vi "Gui_SetupTimingScript_Ions.vi"(8 "error in (no error)":errorcluster, 11 "QMH UI Cluster":T4) -> (0 "error out":errorcluster caption="sortie d'erreur")   [LabVIEW 2018]
uses:
  controls/EXPERT_Inputs.ctl
  controls/DIGIT_5122_Inputs.ctl
  <instrlib>/niScope/Controls/niScope trigger source.ctl
  controls/HSDIO_6541_Inputs.ctl
  <instrlib>/niHSDIO/niHSDIO.llb/niHSDIO_ctl Trigger Source Values (Ring).ctl
  controls/SOFTWARE_Inputs.ctl
  controls/AO_6711_Inputs.ctl
  controls/AWG_5421_Inputs.ctl
  <instrlib>/niFgen/niFgen.llb/niFgen_ctl Trigger Source Values (Ring).ctl
  controls/XML_Inputs.ctl
  controls/SEQUENCE_Inputs.ctl
  controls/EXCIT_Inputs.ctl
  controls/DATA_Inputs.ctl
  controls/TIMING_Inputs.ctl
  controls/PROCESSING_Inputs.ctl
  controls/TRAPPING_Inputs.ctl
  controls/TIMING_Mandatory_Items.ctl
  controls/QMH_UI_Cluster.ctl
  controls/QMH_UI_References.ctl
  controls/QMH_UI_Report.ctl
  controls/QMH_UI_Command.ctl
  controls/QMH_ICR_Command.ctl
  controls/QMH_Status.ctl
  controls/TIMING_Table.ctl
  controls/TIMING_Optional_Items.ctl
panel:
  out "Ouput Script":string
  in  "TIMING Table":T1={"Mandatory Items"={"Script Name"="", "GINI Time Period"=100.0, "HSDIO Delay"=60.0, "Shutter Duration before"=50000.0, "Shutter Duration after"=50000.0, "Filter Tau"=2.0, "Emtyping Duration"=1000.0}, "Optional Items"={"Eject"=0, "Acq"=0, "Excit"=0, "Gas"=0, "Laser"=0, "Lamp"=0}, "Times Table"=[["Excit1", "name", "Swift", "0.5", "1200", "70", "150", "550", "0", "0", "0"]]} {"Optional Items"."Laser" min=0 max=3; "Optional Items"."Gas" min=0 max=5; "Mandatory Items"."GINI Time Period" min=100000.0 max=1000000.0 format="%#_7g"; "Mandatory Items"."Shutter Duration after" min=2.0 max=100000.0; "Mandatory Items"."HSDIO Delay" min=0.0 max=100.0; "Mandatory Items"."Shutter Duration before" min=2.0 max=100000.0; "Mandatory Items"."Filter Tau" min=1000.0 max=2000.0; "Mandatory Items"."Emtyping Duration" min=2.0 format="%#_8g"}
  out "Total Duration (estimation)":i16=1 min=1 max=10 step=1
  in  "Number of Ions Refills":i16=1 min=1 max=100 step=1
  in  "REWRITE HEADER":bool
  in  "Mandatory Items":T2={"Script Name"="ForTestPurpose", "GINI Time Period"=100.0, "HSDIO Delay"=60.0, "Shutter Duration before"=50000.0, "Shutter Duration after"=50000.0, "Filter Tau"=2000.0, "Emtyping Duration"=1000000.0} caption="TIMING Mandatory Items" {"GINI Time Period" min=100000.0 max=1000000.0 format="%#_7g"; "Shutter Duration after" min=2.0 max=100000.0; "HSDIO Delay" min=0.0 max=100.0; "Shutter Duration before" min=2.0 max=100000.0; "Filter Tau" min=1000.0 max=2000.0; "Emtyping Duration" min=2.0 format="%#_8g"}
  in  "SEQUENCE Inputs":T10={"EXCIT Inputs"={"Number of Excitations"=1, "Script Text"="", "Table of Waveforms"=[]}, "DATA Inputs"={"Record Length"=524000, "Sample Rate"=2000000.0, "Data Type"=0, "Vertical Range"=10.0, "Acquisition Duration"=262.0}, "TIMING Inputs"={"Number of Acquisitions "=1, "Number of Accumulations"=1, "Table of Waveforms"=[], "Script Text"=""}, "PROCESSING Inputs"={"Reference Mass"=300.0939, "Cyclotron Freq"=255.727, "Magnetron Freq"=0.001}, "TRAPPING Inputs"={"Number of Channels"=4, "Init Values"=[2.0, 9.0, 2.0, 9.0], "Opening Values"=[0.0, 0.0, 0.0, 0.0], "Trapping Values"=[2.0, 9.0, 2.0, 9.0], "Emptying Values"=[-10.0, -10.0, -10.0, -10.0], "Adiabatic ON"=FALSE, "Adiabatic Duration"=100, "Adiabatic Waveforms"=["Adiabatic_None_2_2_2000", "Adiabatic_Ramp_9_0_2000", "Adiabatic_None_2_2_2000", "Adiabatic_RC_9_0_2000"], "Ions Refill ON"=FALSE, "Number of Ions Refills"=1, "Trapping Delay"=400.0, "Trapping Duration"=300.0}} {"TRAPPING Inputs"."Trapping Duration" min=2.0; "TRAPPING Inputs"."Trapping Delay" min=2.0; "TRAPPING Inputs"."Number of Ions Refills" min=1 max=1000; "TRAPPING Inputs"."Trapping Values" min=-10.0 max=10.0; "TRAPPING Inputs"."Init Values" min=-10.0 max=10.0; "TRAPPING Inputs"."Emptying Values" min=-10.0 max=10.0; "TRAPPING Inputs"."Opening Values" min=-10.0 max=10.0; "PROCESSING Inputs"."Magnetron Freq" format="%.5g"; "PROCESSING Inputs"."Cyclotron Freq" format="%.5g"; "PROCESSING Inputs"."Reference Mass" format="%.5g"; "TIMING Inputs"."Number of Accumulations" min=0 max=50 step=1; "TIMING Inputs"."Number of Acquisitions" min=1 max=10 step=1; "DATA Inputs"."Vertical Range" items=["0.2"=0.2, "0.4"=0.4, "1"=1.0, "2"=2.0, "4"=4.0, "10"=10.0]; "DATA Inputs"."Data Type" items=["I16", "DBL"]; "DATA Inputs"."Sample Rate" items=["1 MHz"=1000000.0, "2 MHz"=2000000.0, "5 MHz"=5000000.0, "10 MHz"=10000000.0, "20 MHz"=20000000.0, "25 MHz"=25000000.0, "50 MHz"=50000000.0, "100 MHz"=100000000.0]; "EXCIT Inputs"."Number of Excitations" min=1 max=10}
  out "Number of Excitations":i16=1 min=1 max=10 step=1
  in  "Number Of Accumulations":i16=1 caption="Number of Accumulations" min=0 max=50 step=1
  out "Number of Acquisitions":i16=1 min=1 max=10 step=1
  in  "OK":bool
  in  "CHECK":bool
  in  "EXPERT Inputs":T16={"DIGIT 5122 Inputs"={"Sample Rate"=10000.0, "Resource Name"="DIGIT_5122", "Channel Name"="0", "Trigger Source"="VAL_EXTERNAL", "Vertical Range"=10.0, "Trigger Level"=3.0}, "HSDIO 6541 Inputs"={"Resource Name"="HSDIO_6541", "Clock Rate"=1000000.0, "Trigger Source"="PFI0"}, "SOFTWARE Inputs"={"Application Directory"=path "D:/S.O.F.T.S/LABVIEW/PIL", "Software Version"="1.0.0", "Data Path"=path "D:/PIRENEA/DATA", "XML Path"=path "D:/PIRENEA/DATA", "XML File Filter"="*.xml", "XML Saved Path"=path "D:/PIRENEA/DATA/SAVED", "Excit Scripts Path"=path "D:/PIRENEA/EXCIT_SCRIPTS", "Excit Scripts File Filter"="*.txt", "Excit Waveforms Path"=path "D:/PIRENEA/EXCIT_WFMS", "Excit Waveforms File Filter"="*.bin", "Timing Scripts Path"=path "D:/PIRENEA/TECHNICAL/TIMING_SCRIPTS", "Timing Scripts File Filter"="*.txt", "Timing Waveforms Path"=path "D:/PIRENEA/TECHNICAL/TIMING_WFMS", "Timing Waveforms File Filter"="*.bin", "Trapping Waveforms Path"=path "D:/PIRENEA/TRAPPING_WFMS", "Trapping Waveforms File Filter"="*.bin"}, "AO 6711 Inputs"={"Physical Channels"="AO_6711/ao0:3", "Min Voltage"=-10.0, "Max Voltage"=10.0, "Trigger Source"="/AO_6711/PFI3", "Counter"="AO_6711/ctr0"}, "AWG 5421 Inputs"={"Resource Name"="AWG_5421", "Sample Rate"=10000000.0, "Trigger Type"=2, "Trigger Source"="PFI0", "Waveform Gain"=0.31, "Digital Filter ON"=TRUE}, "XML Inputs"={"Version Tag Name"="XML_Version", "Version String"="1.0"}} {"AWG 5421 Inputs"."Sample Rate" format="%.2p"; "AWG 5421 Inputs"."Trigger Type" items=["None", "Software Edge", "Digital Edge", "Digital Level"]; "AO 6711 Inputs"."Max Voltage" min=-10.0 max=10.0; "AO 6711 Inputs"."Min Voltage" min=-10.0 max=10.0; "HSDIO 6541 Inputs"."Clock Rate" format="%.2p"; "DIGIT 5122 Inputs"."Trigger Level" format="%.2f"; "DIGIT 5122 Inputs"."Vertical Range" format="%.2f"; "DIGIT 5122 Inputs"."Sample Rate" step=65535.0 format="%#_3p"}
  in  "LOAD":bool
  in  "Timing Script":string
  # "GO_out"
  # "Gout"
  # "GI_in"
  # "Gin"
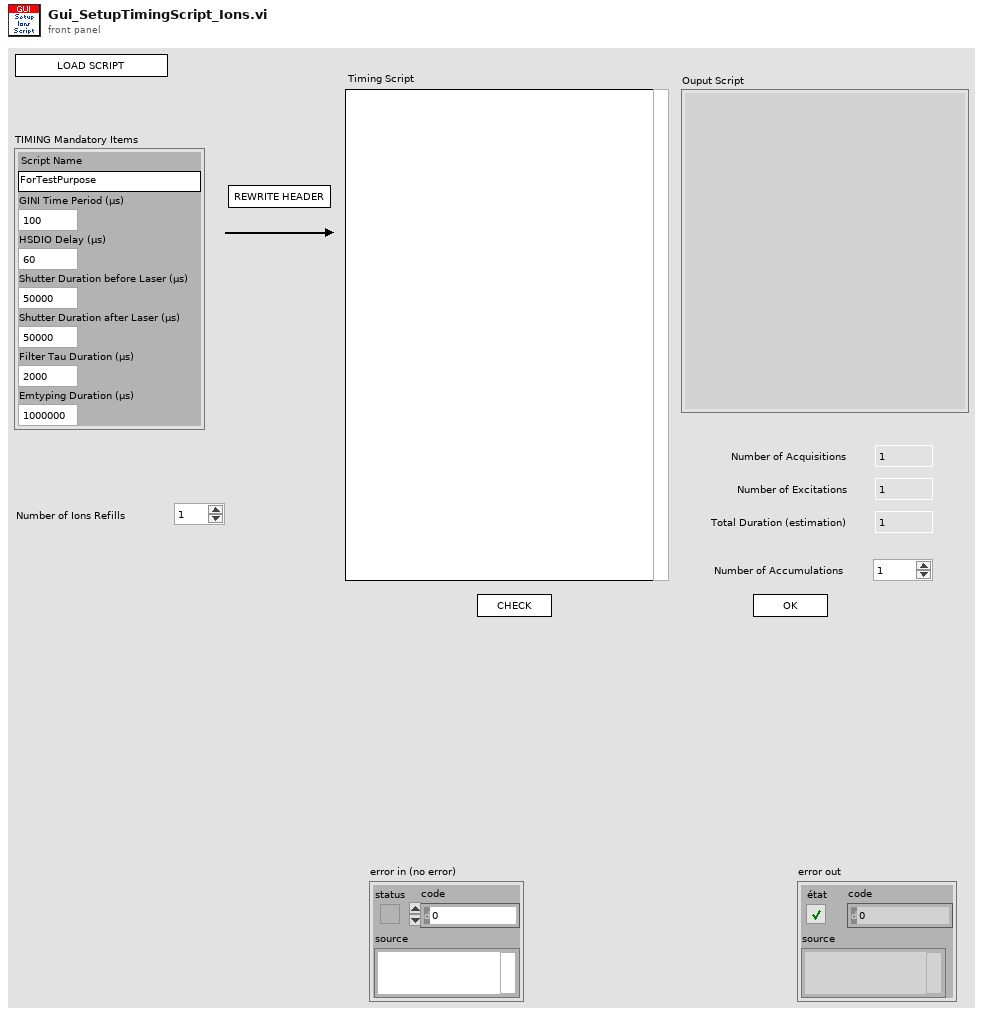
[diagram p1: front panel]
types:
  T1 = typedef "TIMING_Table.ctl" = cluster{"Mandatory Items":T2, "Optional Items":T3, "Times Table":string[][]}
  T2 = typedef "TIMING_Mandatory_Items.ctl" = cluster{"Script Name":string, "GINI Time Period":dbl, "HSDIO Delay":dbl, "Shutter Duration before":dbl, "Shutter Duration after":dbl, "Filter Tau":dbl, "Emtyping Duration":dbl}
  T3 = typedef "TIMING_Optional_Items.ctl" = cluster{"Eject":u32, "Acq":i32, "Excit":u32, "Gas":i32, "Laser":i32, "Lamp":i32}
  T4 = typedef "QMH_UI_Cluster.ctl" = cluster{"QMH UI References":T5, "QMH UI Report":T6}
  T5 = typedef "QMH_UI_References.ctl" = cluster{"Refnum Load":refnum<vi>, "Refnum Save As":refnum<vi>, "Refnum Start":refnum<vi>, "Refnum Exit":refnum<vi>, "Refnum Tabs":refnum<vi>, "Refnum SPECTRUM":refnum<vi>, "Refnum EXPERIMENT":refnum<vi>, "Refnum VOLTAGES":refnum<vi>, "Refnum SEQUENCE":refnum<vi>, "Refnum EXPERT":refnum<vi>, "Refnum EXCIT Table":refnum<vi>, "Refnum TIMING Table":refnum<vi>, "Refnum CHANGE Experiment":refnum<vi>, "Refnum CHANGE Voltages":refnum<vi>, "Refnum CHANGE Sequence":refnum<vi>, "Refnum CHANGE Expert":refnum<vi>, "Refnum CHANGE Scientist":refnum<vi>, "Refnum PIL Status":refnum<vi>}
  T6 = typedef "QMH_UI_Report.ctl" = cluster{"UI Status":T7, "ICR Status":T8, "QMH Status":T9}
  T7 = typedef "QMH_UI_Command.ctl" = enum16{"Initialize", "UI Load", "UI Save", "UI Save As", "UI Change Experiment", "UI Change Voltages", "UI Change Sequence", "UI Change Expert", "UI Change Scientist", "Ready to Start", "UI Start", "Waiting for ICR", "UI Exit", "Update Report", "Update ICR Status", "Waiting for User"}
  T8 = typedef "QMH_ICR_Command.ctl" = enum16{"Initialize", "Sequence Setup", "ICR Start", "ICR Stop", "Hardware Setup", "Next Accumulation", "Waiting for Trigger", "Sequence Started", "Sequence Finished", "Writing Data", "Hardware Reset", "Exit"}
  T9 = typedef "QMH_Status.ctl" = enum16{"Init", "Loading", "Setup", "Ready to Start", "Started", "Idle"}
  T10 = typedef "SEQUENCE_Inputs.ctl" = cluster{"EXCIT Inputs":T11, "DATA Inputs":T12, "TIMING Inputs":T13, "PROCESSING Inputs":T14, "TRAPPING Inputs":T15}
  T11 = typedef "EXCIT_Inputs.ctl" = cluster{"Number of Excitations":i32, "Script Text":string, "Table of Waveforms":string[]}
  T12 = typedef "DATA_Inputs.ctl" = cluster{"Record Length":i32, "Sample Rate":dbl, "Data Type":u8, "Vertical Range":dbl, "Acquisition Duration":dbl}
  T13 = typedef "TIMING_Inputs.ctl" = cluster{"Number of Acquisitions ":i16, "Number of Accumulations":i16, "Table of Waveforms":string[], "Script Text":string}
  T14 = typedef "PROCESSING_Inputs.ctl" = cluster{"Reference Mass":dbl, "Cyclotron Freq":dbl, "Magnetron Freq":dbl}
  T15 = typedef "TRAPPING_Inputs.ctl" = cluster{"Number of Channels":i32, "Init Values":dbl[], "Opening Values":dbl[], "Trapping Values":dbl[], "Emptying Values":dbl[], "Adiabatic ON":bool, "Adiabatic Duration":i32, "Adiabatic Waveforms":string[], "Ions Refill ON":bool, "Number of Ions Refills":i32, "Trapping Delay":dbl, "Trapping Duration":dbl}
  T16 = typedef "EXPERT_Inputs.ctl" = cluster{"DIGIT 5122 Inputs":T17, "HSDIO 6541 Inputs":T19, "SOFTWARE Inputs":T21, "AO 6711 Inputs":T22, "AWG 5421 Inputs":T23, "XML Inputs":T25}
  T17 = typedef "DIGIT_5122_Inputs.ctl" = cluster{"Sample Rate":dbl, "Resource Name":refnum<k15>, "Channel Name":string, "Trigger Source":T18, "Vertical Range":dbl, "Trigger Level":dbl}
  T18 = typedef "niScope trigger source.ctl" = string
  T19 = typedef "HSDIO_6541_Inputs.ctl" = cluster{"Resource Name":refnum<k15>, "Clock Rate":dbl, "Trigger Source":T20}
  T20 = typedef "niHSDIO_ctl Trigger Source Values (Ring).ctl" = string
  T21 = typedef "SOFTWARE_Inputs.ctl" = cluster{"Application Directory":path, "Software Version":string, "Data Path":path, "XML Path":path, "XML File Filter":string, "XML Saved Path":path, "Excit Scripts Path":path, "Excit Scripts File Filter":string, "Excit Waveforms Path":path, "Excit Waveforms File Filter":string, "Timing Scripts Path":path, "Timing Scripts File Filter":string, "Timing Waveforms Path":path, "Timing Waveforms File Filter":string, "Trapping Waveforms Path":path, "Trapping Waveforms File Filter":string}
  T22 = typedef "AO_6711_Inputs.ctl" = cluster{"Physical Channels":tag, "Min Voltage":dbl, "Max Voltage":dbl, "Trigger Source":tag, "Counter":tag}
  T23 = typedef "AWG_5421_Inputs.ctl" = cluster{"Resource Name":refnum<k15>, "Sample Rate":dbl, "Trigger Type":u16, "Trigger Source":T24, "Waveform Gain":dbl, "Digital Filter ON":bool}
  T24 = typedef "niFgen_ctl Trigger Source Values (Ring).ctl" = string
  T25 = typedef "XML_Inputs.ctl" = cluster{"Version Tag Name":string, "Version String":string}
  T26 = enum16{"Native", "Native Command Line", "UNIX", "Macintosh", "DOS"}
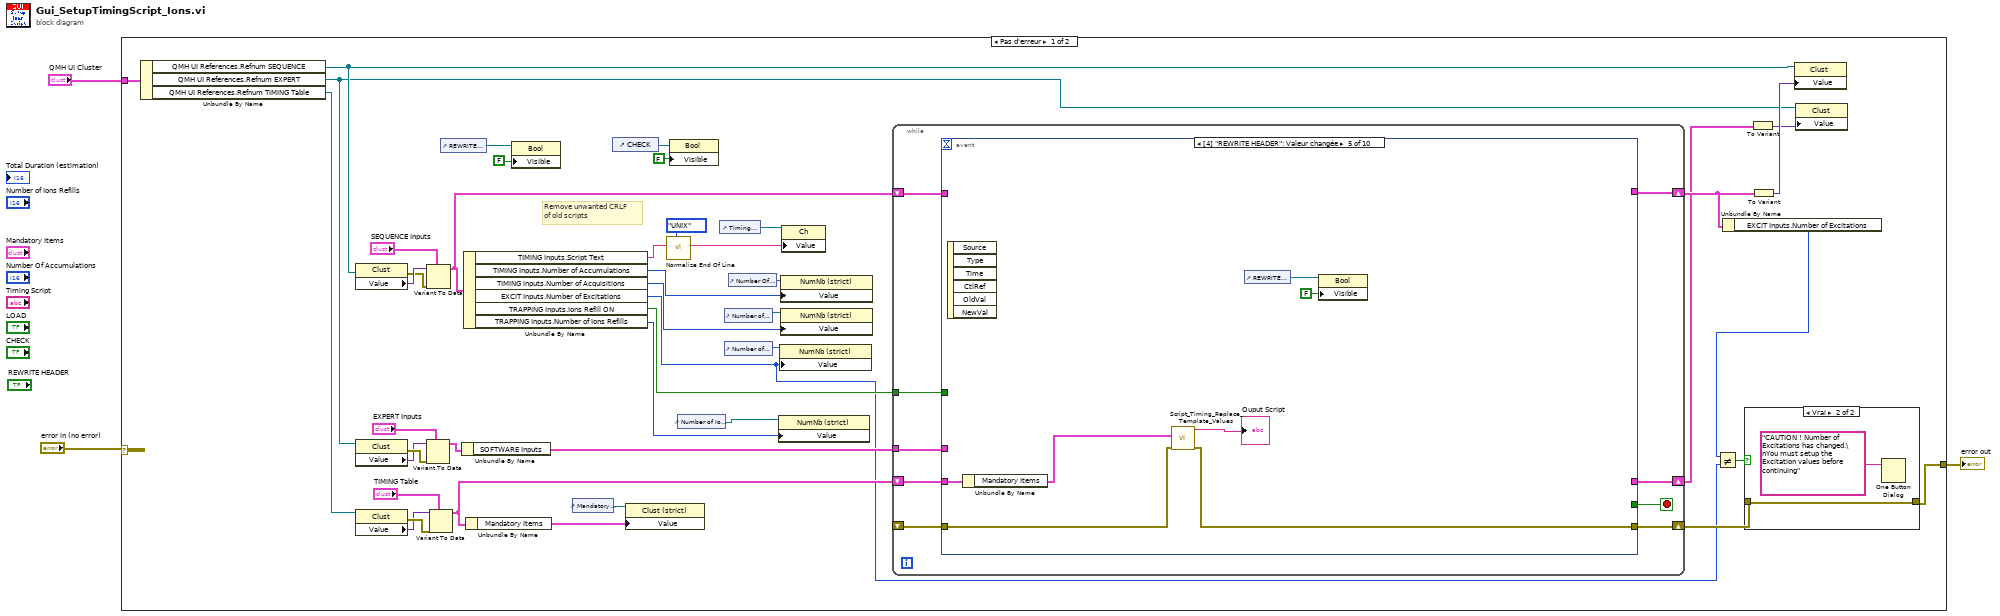
[diagram p0: block diagram]
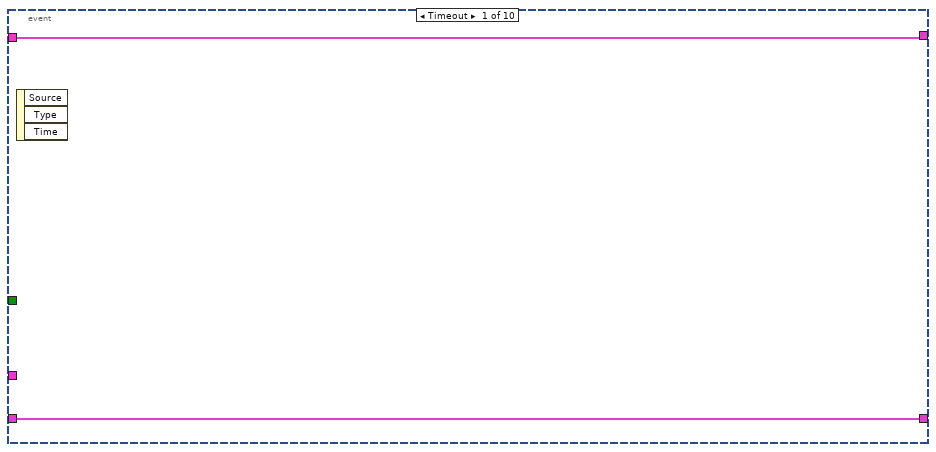
[diagram p3: hidden frame]
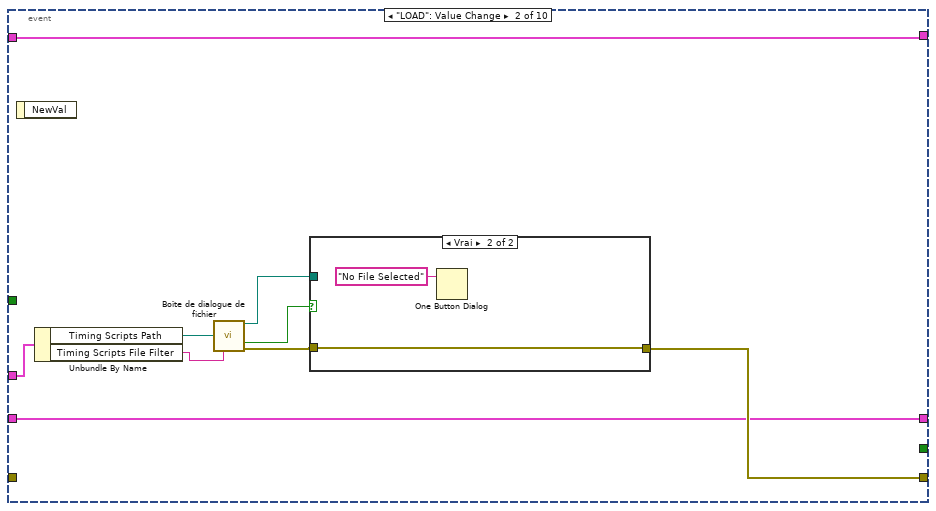
[diagram p4: hidden frame]
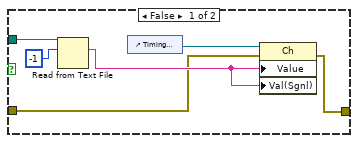
[diagram p5: hidden frame]
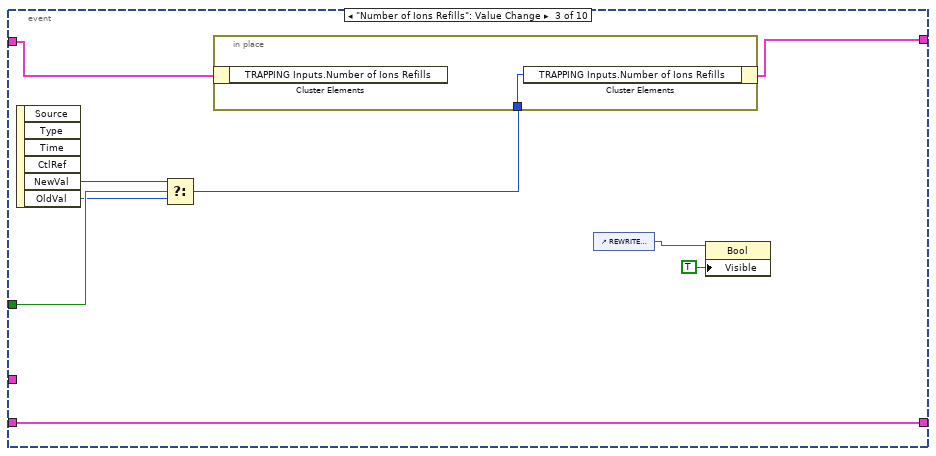
[diagram p6: hidden frame]
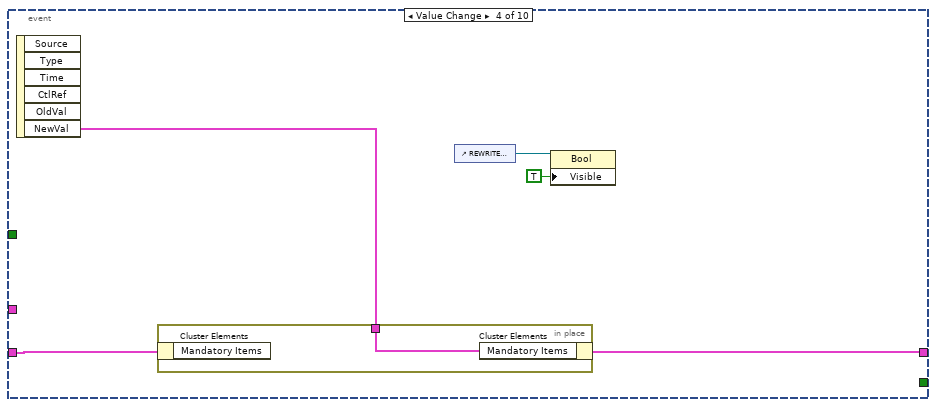
[diagram p7: hidden frame]
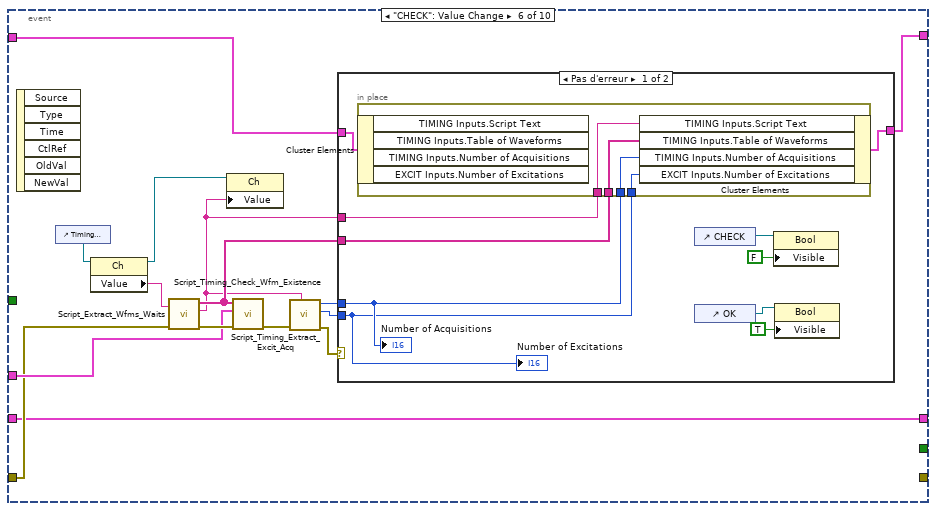
[diagram p8: hidden frame]
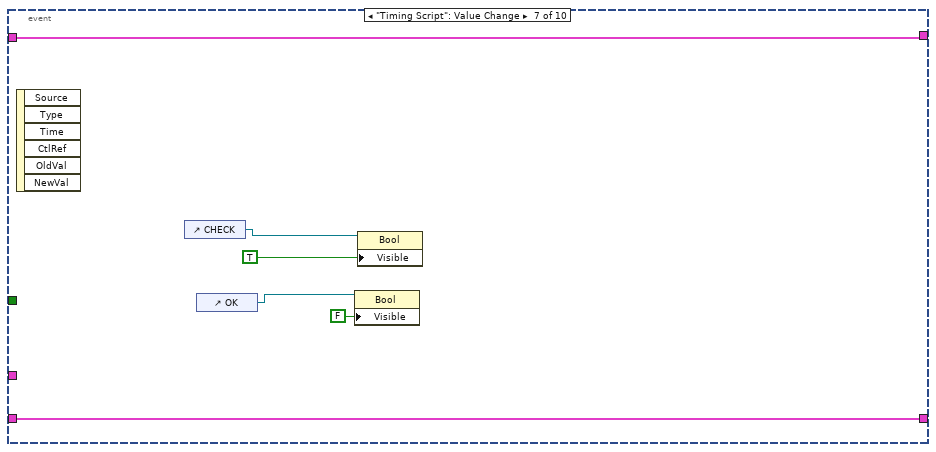
[diagram p10: hidden frame]
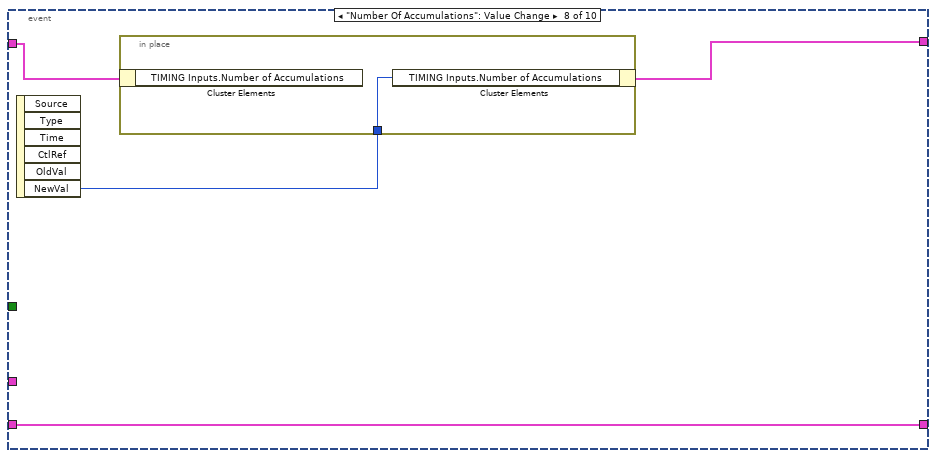
[diagram p11: hidden frame]
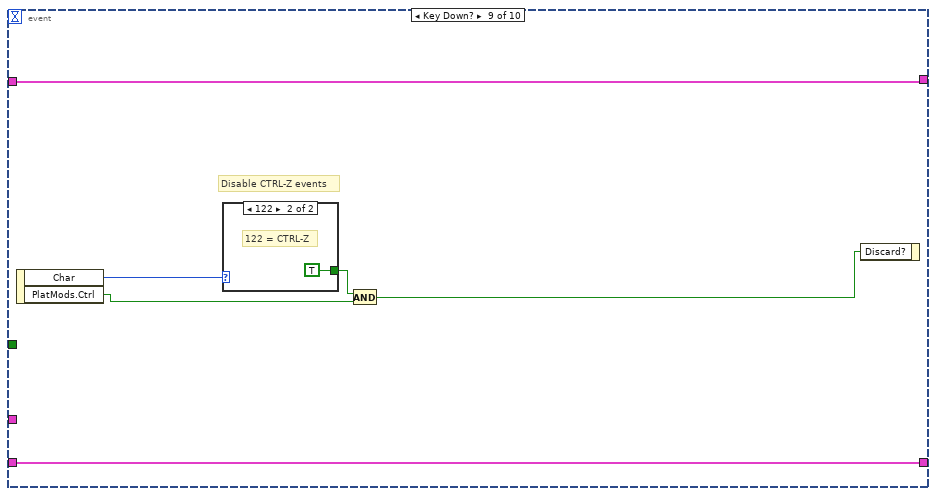
[diagram p12: hidden frame]
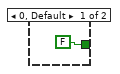
[diagram p13: hidden frame]
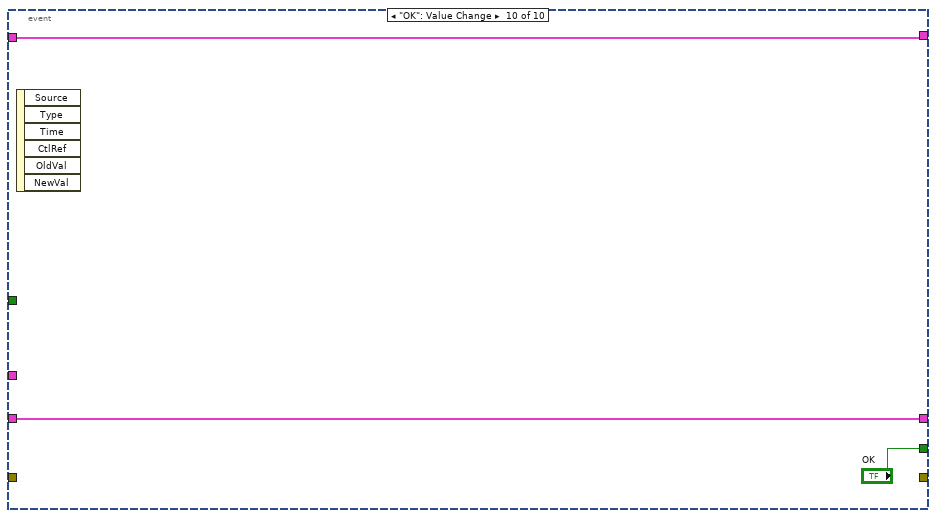
[diagram p14: hidden frame]
diagram:
  n1 = case shown="Pas d'erreur" "error in (no error)" {
    selector: "error in (no error)" -> [_ w154]
    tunnel: [w37 w154] -> w2
    tunnel: "QMH UI Cluster" -> [w34 _]
    frame No Error {
      # "Remove unwanted CRLF\nof old scripts"
      n2 = Unbundle By Name(w34) -> ("QMH UI References.Refnum SEQUENCE"=w14:refnum<vi>, "QMH UI References.Refnum EXPERT"=w7:refnum<vi>, "QMH UI References.Refnum TIMING Table"=w22:refnum<vi>)
      n3 = property class="Clust"(reference=w14) -> (error out=w15:errorcluster, "Value"=w33:variant)  [unwired: 1 in, 1 out]
      n4 = property class="Clust"(reference=w7) -> (error out=w27:errorcluster, "Value"=w24:variant)  [unwired: 1 in, 1 out]
      n5 = property class="Clust"(reference=w22) -> (error out=w26:errorcluster, "Value"=w25:variant)  [unwired: 1 in, 1 out]
      n6 = Variant To Data(error in=w27, type="EXPERT Inputs", Variant=w24) -> (data=w40:T16)  [unwired: 1 out]
      n7 = Variant To Data(error in=w15, type="SEQUENCE Inputs", Variant=w33) -> (data=w18:T10)  [unwired: 1 out]
      n8 = Variant To Data(error in=w26, type="TIMING Table", Variant=w25) -> (data=w13:T1)  [unwired: 1 out]
      n9 = control-ref of="REWRITE HEADER"() -> (w5:refnum<vi>)
      n10 = Unbundle By Name(w40) -> ("SOFTWARE Inputs"=w46:T21)
      n11 = Unbundle By Name(w18) -> ("TIMING Inputs.Script Text"=w31:string, "TIMING Inputs.Number of Accumulations"=w30:i16, "TIMING Inputs.Number of Acquisitions"=w29:i16, "EXCIT Inputs.Number of Excitations"=w9:i32, "TRAPPING Inputs.Ions Refill ON"=w10:bool, "TRAPPING Inputs.Number of Ions Refills"=w11:i32)
      n12 = Unbundle By Name(w13) -> ("Mandatory Items"=w20:T2)
      n13 = property class="Bool"(reference=w5, "Visible"=FALSE) -> ()  [unwired: 1 in, 2 out]
      n14 = control-ref of="Mandatory Items"() -> (w21:refnum<vi>)
      n15 = control-ref of="CHECK"() -> (w44:refnum<vi>)
      n16 = property class="Clust (strict)"(reference=w21, "Value"=w20) -> ()  [unwired: 1 in, 2 out]
      n17 = call <vilib>:"Normalize End Of Line.vi"("end of line (Native)"=T26."UNIX", "string in"=w31) -> ("string out"=w35:string)  [unwired: 6 in]
      n18 = property class="Bool"(reference=w44, "Visible"=FALSE) -> ()  [unwired: 1 in, 2 out]
      n19 = control-ref of="Number of Ions Refills"() -> (w12:refnum<vi>)
      n20 = control-ref of="Timing Script"() -> (w47:refnum<vi>)
      n21 = control-ref of="Number of Acquisitions"() -> (w42:refnum<vi>)
      n22 = control-ref of="Number of Excitations"() -> (w41:refnum<vi>)
      n23 = control-ref of="Number Of Accumulations"() -> (w43:refnum<vi>)
      n24 = property class="NumNb (strict)"(reference=w12, "Value"=w11) -> ()  [unwired: 1 in, 2 out]
      n25 = property class="NumNb (strict)"(reference=w41, "Value"=w9) -> ()  [unwired: 1 in, 2 out]
      n26 = property class="NumNb (strict)"(reference=w43, "Value"=w30) -> ()  [unwired: 1 in, 2 out]
      n27 = property class="NumNb (strict)"(reference=w42, "Value"=w29) -> ()  [unwired: 1 in, 2 out]
      n28 = property class="Ch"(reference=w47, "Value"=w35) -> ()  [unwired: 1 in, 2 out]
      n29 = while {
        shift-right: [w57] -> w38
        shift-left: _ -> [w59]
        tunnel: w46 -> [w54]
        shift-right: [w55] -> w17
        shift-left: w18 -> [w56]
        shift-right: [w51] -> w8
        shift-left: w13 -> [w53]
        tunnel: w10 -> [w52]
        stop <- w58 stop-if-true
        n30 = event shown="[4] \"REWRITE HEADER\": Valeur changée" {
          selector: _ -> [_ _ _ _ _ _ _ _ _ _]
          dyn-events: _ -> [_ _ _ _ _ _ _ _ _ _]
          timeout: _ -> [_ _ _ _ _ _ _ _ _ _]
          tunnel: w59 -> [_ _ _ _ w99 w103 _ _ _ _]
          tunnel: [_ w66 _ _ w98 _ _ _ _ _] -> w57
          tunnel: [_ _ _ _ _ _ _ _ _ "OK"] -> w58
          tunnel: w56 -> [w61 w67 w87 _ _ w114 w135 w139 w144 w152]
          tunnel: [w61 w67 w86 _ _ w113 w135 w140 w144 w152] -> w55
          tunnel: w54 -> [_ w65 _ _ _ w111 _ _ _ _]
          tunnel: w53 -> [w60 w62 w81 w93 w97 w102 w132 w138 w143 w151]
          tunnel: w52 -> [_ _ w85 _ _ _ _ _ _ _]
          tunnel: [w60 w62 w81 w91 _ w102 w132 w138 w143 w151] -> w51
          event Timeout {
            n31 = event-data() -> ()  [unwired: 1 in, 3 out]
          }
          event "LOAD": Value Change {
            n32 = event-data() -> ()  [unwired: 1 in, 1 out]
            n33 = Unbundle By Name(w65) -> ("Timing Scripts Path"=w63:path, "Timing Scripts File Filter"=w64:string)
            n34 = call "Boîte de dialogue de fichier"("start path"=w63, "pattern (all files)"=w64) -> ("selected path"=w70:path, "cancelled"=w69:bool, "error out"=w68:errorcluster)  [unwired: 10 in, 1 out]
            n35 = case shown="Vrai" w69 {
              tunnel: w70 -> [w76 _]
              tunnel: w68 -> [w72 w77]
              tunnel: [w71 w77] -> w66
              frame False {
                n36 = Read from Text File(file (use dialog)=w76, count=-1 ("nombre")) -> (text=w73:string)  [unwired: 2 in, 3 out]
                n37 = control-ref of="Timing Script"() -> (w74:refnum<vi>)
                n38 = property class="Ch"(reference=w74, error in=w72, "Value"=w73, "Val(Sgnl)"=w73) -> (error out=w71:errorcluster)  [unwired: 1 out]
              }
              frame True {
                n39 = One Button Dialog(message="No File Selected") -> ()  [unwired: 1 in, 1 out]
              }
            }
          }
          event "Number of Ions Refills": Value Change {
            n40 = event-data() -> ("NewVal"=w84:i16, "OldVal"=w83:i16)  [unwired: 1 in, 4 out]
            n41 = Select(t=w84, s=w85, f=w83) -> (s? t:f=w82:i16)
            n42 = in-place {
              in-place-border: w82 -> [w88]
              n43 = in-place-cluster #1(w87) -> ()  [unwired: 1 out]
              n44 = in-place-cluster #1("TRAPPING Inputs.Number of Ions Refills"=w88) -> (w86:T10)
            }
            n45 = control-ref of="REWRITE HEADER"() -> (w80:refnum<vi>)
            n46 = property class="Bool"(reference=w80, "Visible"=TRUE) -> ()  [unwired: 1 in, 2 out]
          }
          event Value Change {
            n47 = event-data() -> ("NewVal"=w92:T2)  [unwired: 1 in, 5 out]
            n48 = in-place {
              in-place-border: w92 -> [w94]
              n49 = in-place-cluster #2(w93) -> ()  [unwired: 1 out]
              n50 = in-place-cluster #2("Mandatory Items"=w94) -> (w91:T1)
            }
            n51 = control-ref of="REWRITE HEADER"() -> (w90:refnum<vi>)
            n52 = property class="Bool"(reference=w90, "Visible"=TRUE) -> ()  [unwired: 1 in, 2 out]
          }
          event "REWRITE HEADER": Value Change {
            n53 = event-data() -> ()  [unwired: 1 in, 6 out]
            n54 = Unbundle By Name(w97) -> ("Mandatory Items"=w96:T2)
            n55 = call "Script_Timing_Replace_Template_Values.vi"("error in (no error)"=w99, "Mandatory Items"=w96) -> ("error out"=w98:errorcluster, "Ouput Script"=→"Ouput Script":string)  [unwired: 8 in]
            n56 = control-ref of="REWRITE HEADER"() -> (w100:refnum<vi>)
            n57 = property class="Bool"(reference=w100, "Visible"=FALSE) -> ()  [unwired: 1 in, 2 out]
          }
          event "CHECK": Value Change {
            n58 = event-data() -> ()  [unwired: 1 in, 6 out]
            n59 = control-ref of="Timing Script"() -> (w116:refnum<vi>)
            n60 = property class="Ch"(reference=w116) -> (reference out=w104:refnum<vi>, "Value"=w108:string)  [unwired: 1 in, 1 out]
            n61 = call "Script_Extract_Wfms_Waits.vi"("Script Text"=w108, "error in (no error)"=w103) -> ("error out"=w115:errorcluster, "Script Text Cleaned"=w105:string, "Table of Loaded Wfms"=w112:string[])  [unwired: 6 in, 1 out]
            n62 = property class="Ch"(reference=w104, "Value"=w105) -> ()  [unwired: 1 in, 2 out]
            n63 = call "Script_Timing_Check_Wfm_Existence.vi"("error  in"=w115, "SOFTWARE Inputs"=w111, "Table of Waveforms"=w112) -> ("error out"=w110:errorcluster)  [unwired: 8 in]
            n64 = call "Script_Timing_Extract_Excit_Acq.vi"("Script Text"=w105, "error in (no error)"=w110) -> ("error out"=w109:errorcluster, "Number of Excits"=w106:i16, "Number of Acqs"=w107:i16)  [unwired: 7 in]
            n65 = case shown="Pas d'erreur" w109 {
              tunnel: w114 -> [w117 w131]
              tunnel: [w124 w131] -> w113
              tunnel: w105 -> [w123 _]
              tunnel: w112 -> [w122 _]
              tunnel: w107 -> [w121 _]
              tunnel: w106 -> [w120 _]
              frame No Error {
                n66 = in-place {
                  in-place-border: w123 -> [w130]
                  in-place-border: w122 -> [w129]
                  in-place-border: w121 -> [w128]
                  in-place-border: w120 -> [w127]
                  n67 = in-place-cluster #3(w117) -> ()  [unwired: 4 out]
                  n68 = in-place-cluster #3("TIMING Inputs.Script Text"=w130, "TIMING Inputs.Table of Waveforms"=w129, "TIMING Inputs.Number of Acquisitions"=w128, "EXCIT Inputs.Number of Excitations"=w127) -> (w124:T10)
                }
                n69 = control-ref of="CHECK"() -> (w126:refnum<vi>)
                n70 = control-ref of="OK"() -> (w119:refnum<vi>)
                n71 = property class="Bool"(reference=w126, "Visible"=FALSE) -> ()  [unwired: 1 in, 2 out]
                n72 = property class="Bool"(reference=w119, "Visible"=TRUE) -> ()  [unwired: 1 in, 2 out]
                "Number of Acquisitions" <- w121
                "Number of Excitations" <- w120
              }
              frame Error {
              }
            }
          }
          event "Timing Script": Value Change {
            n73 = event-data() -> ()  [unwired: 1 in, 6 out]
            n74 = control-ref of="CHECK"() -> (w137:refnum<vi>)
            n75 = control-ref of="OK"() -> (w134:refnum<vi>)
            n76 = property class="Bool"(reference=w134, "Visible"=FALSE) -> ()  [unwired: 1 in, 2 out]
            n77 = property class="Bool"(reference=w137, "Visible"=TRUE) -> ()  [unwired: 1 in, 2 out]
          }
          event "Number Of Accumulations": Value Change {
            n78 = event-data() -> ("NewVal"=w141:i16)  [unwired: 1 in, 5 out]
            n79 = in-place {
              in-place-border: w141 -> [w142]
              n80 = in-place-cluster #4(w139) -> ()  [unwired: 1 out]
              n81 = in-place-cluster #4("TIMING Inputs.Number of Accumulations"=w142) -> (w140:T10)
            }
          }
          event Key Down? {
            # "Disable CTRL-Z events"
            n82 = event-data() -> ("Char"=w147:i16, "PlatMods.Ctrl"=w146:bool)  [unwired: 1 in]
            n83 = case shown="122" w147 {
              tunnel: [FALSE TRUE] -> w148
              frame 0, Default {
              }
              frame 122 {
                # "122 = CTRL-Z"
              }
            }
            n84 = And(x=w148, y=w146) -> (x .and. y?=w145:bool)
            n85 = event-data("Discard?"=w145) -> ()  [unwired: 1 in, 1 out]
          }
          event "OK": Value Change {
            n86 = event-data() -> ()  [unwired: 1 in, 6 out]
          }
        }
      }
      n87 = Unbundle By Name(w17) -> ("EXCIT Inputs.Number of Excitations"=w19:i32)
      n88 = Not Equal?(x=w19, y=w9) -> (x != y?=w39:bool)
      n89 = case shown="Vrai" w39 {
        tunnel: w38 -> [w48 w49]
        tunnel: [w48 w49] -> w37
        frame False {
        }
        frame True {
          n90 = One Button Dialog(message="CAUTION ! Number of Excitations has changed.\nYou must setup the Excitation values before continuing") -> ()  [unwired: 1 in, 1 out]
        }
      }
      n91 = To Variant(anything=w8) -> (Variant=w6:variant)
      n92 = To Variant(anything=w17) -> (Variant=w16:variant)
      n93 = property class="Clust"(reference=w14, "Value"=w16) -> ()  [unwired: 1 in, 2 out]
      n94 = property class="Clust"(reference=w7, "Value"=w6) -> ()  [unwired: 1 in, 2 out]
    }
    frame Error {
    }
  }
  "error out" <- w2
